vi "Change Color Popup.vi"(8 "error in":errorcluster, 11 "Color Value In":u32) -> (0 "error out":errorcluster, 3 "Color Value Out":u32)   [LabVIEW 2019]
doc: "All Rights Reserved © 2017 SyncSols"
uses:
  <vilib>/Utility/inputDevices.llb/keyboardAcquire.vi
panel:
  in  "Select Color":u32(colorbox)
  # "<<Enter to Save the Changes>>"
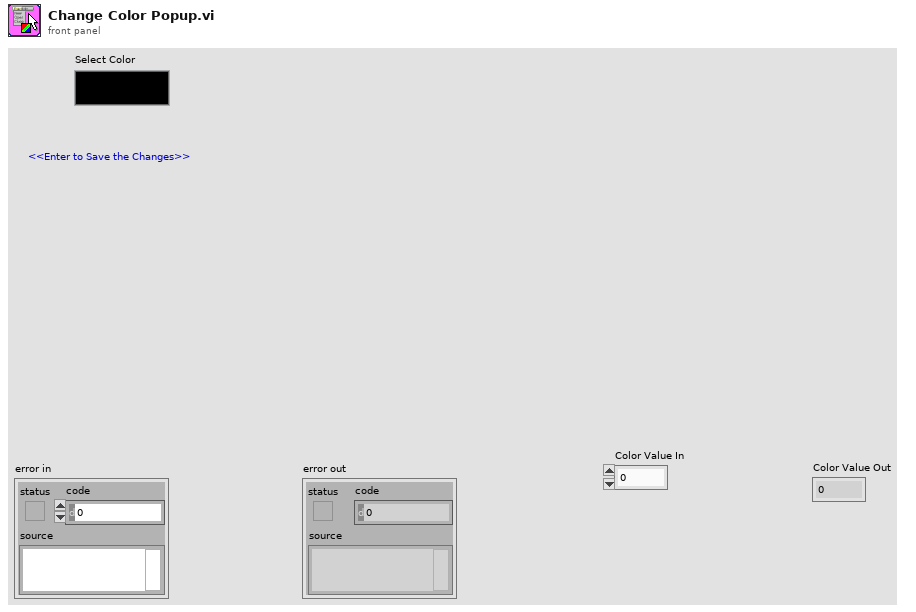
[diagram p1: front panel]
types:
  T1 = enum16{"0", "1", "2", "3", "4", "5", "6", "7", "8", "9", "A", "B", "C", "D", "E", "F", "G", "H", "I", "J", "K", "L", "M", "N", "O", "P", "Q", "R", "S", "T", "U", "V", "W", "X", "Y", "Z", "F1", "F2", "F3", "F4", "F5", "F6", "F7", "F8", "F9", "F10", "F11", "F12", "F13", "F14", "F15", "ADD", "BACK", "BACKSLASH", "CAPITAL", "COMMA", "DECIMAL", "DELETE", "DIVIDE", "DOWN", "END", "EQUALS", "ESCAPE", "GRAVE (`)", "HOME", "INSERT", "LBRACKET", "LCONTROL", "LEFT", "L ALT", "LSHIFT", "LWIN", "MINUS", "MULTIPLY", "NEXT", "NUMLOCK", "NUMPAD_0", "NUMPAD_1", "NUMPAD_2", "NUMPAD_3", "NUMPAD_4", "NUMPAD_5", "NUMPAD_6", "NUMPAD_7", "NUMPAD_8", "NUMPAD_9", "PAUSE", "PERIOD", "PRIOR (PG UP)", "RBRACKET", "RCONTROL", "RETURN", "RIGHT", "R ALT", "RSHIFT", "RWIN", "SCROLL", "SEMICOLON", "SLASH", "SPACE", "SUBTRACT", "TAB", "UP", "ENTER (num pad)", "' (quote)"}
  T2 = enum16{"0", "1", "2", "3", "4", "5", "6", "7", "8", "9", "A", "B", "C", "D", "E", "F", "G", "H", "I", "J", "K", "L", "M", "N", "O", "P", "Q", "R", "S", "T", "U", "V", "W", "X", "Y", "Z", "F1", "F2", "F3", "F4", "F5", "F6", "F7", "F8", "F9", "F10", "F11", "F12", "F13", "F14", "F15", "ADD", "BACK", "BACKSLASH", "CAPITAL", "COMMA", "DECIMAL", "DELETE", "DIVIDE", "DOWN", "END", "EQUALS", "ESCAPE", "GRAVE (`)", "HOME", "INSERT", "LBRACKET", "LCONTROL", "LEFT", "L ALT", "LSHIFT", "LWIN", "MINUS", "MULTIPLY", "NEXT", "NUMLOCK", "NUMPAD_0", "NUMPAD_1", "NUMPAD_2", "NUMPAD_3", "NUMPAD_4", "NUMPAD_5", "NUMPAD_6", "NUMPAD_7", "NUMPAD_8", "NUMPAD_9", "PAUSE", "PERIOD", "PRIOR (PG UP)", "RBRACKET", "RCONTROL", "RETURN", "RIGHT", "R ALT", "RSHIFT", "RWIN", "SCROLL", "SEMICOLON", "SLASH", "SPACE", "SUBTRACT", "TAB", "UP", "ENTER (num pad)", "' (quote)"}[]
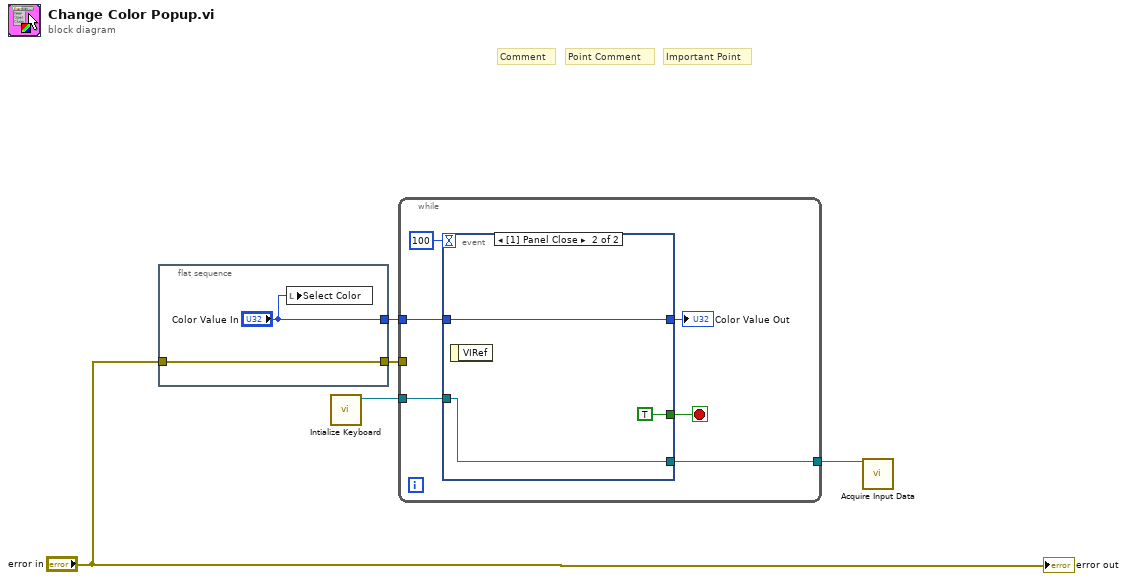
[diagram p0: block diagram]
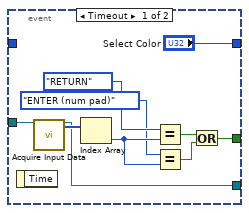
[diagram p2: hidden frame]
diagram:
  # "Important Point"
  # "Point Comment"
  # "Comment"
  n1 = flat-sequence {
    tunnel: [w7] -> w5
    tunnel: "error in" -> [w7]
    tunnel: ["Color Value In"] -> w3
    frame #0 {
      n2 = local write "Select Color"("Color Value In") -> ()
    }
  }
  n3 = call <vilib>:"Intialize Keyboard.vi"() -> ("device ID"=w2:refnum<k1>)  [unwired: 10 in, 1 out]
  n4 = while {
    tunnel: w5 -> [_]
    tunnel: w3 -> [w10]
    tunnel: w2 -> [w9]
    tunnel: [w8] -> w1
    stop <- w11 stop-if-true
    n5 = event shown="[1] Panel Close" {
      selector: _ -> [_ _]
      dyn-events: _ -> [_ _]
      timeout: 100 -> [_ _]
      tunnel: ["Select Color" w25] -> w13
      tunnel: [w17 TRUE] -> w11
      tunnel: w10 -> [_ w25]
      tunnel: w9 -> [w22 w24]
      tunnel: [w14 w24] -> w8
      event Timeout {
        n6 = event-data() -> ()  [unwired: 1 in, 1 out]
        n7 = call-poly <vilib>:"Acquire Input Data.vi"("device ID"=w22) -> ("device ID"=w14:refnum<k1>, "keys pressed"=w21:T2)  [unwired: 16 in, 1 out]
        n8 = Index Array(array=w21) -> (element=w19:T1)  [unwired: 1 in]
        n9 = Equal?(x=T1."RETURN" ("keyType 3"), y=w19) -> (x = y?=w16:bool)
        n10 = Equal?(x=T1."ENTER (num pad)" ("keyType 3"), y=w19) -> (x = y?=w15:bool)
        n11 = Or(x=w16, y=w15) -> (x .or. y?=w17:bool)
      }
      event Panel Close {
        n12 = event-data() -> ()  [unwired: 1 in, 1 out]
      }
    }
    "Color Value Out" <- w13
  }
  n13 = call-poly <vilib>:"Acquire Input Data.vi"("device ID"=w1) -> ()  [unwired: 16 in, 3 out]
  "error out" <- "error in"
